vi "create.vi"(8 "error in (no error)":errorcluster, 10 "handle":i32, 11 "client":i32) -> (0 "error out":errorcluster, 3 "DatasetCreateStaging":refnum<class "DatasetCreateStaging.lvclass">)   [LabVIEW 2020, in "DatasetCreateStaging.lvclass"]
uses:
  DatasetCreateStaging.lvclass
  DatasetCreateStaging.lvclass/DatasetCreateStaging.ctl
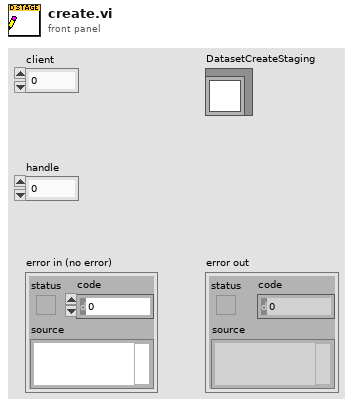
[diagram p1: front panel]
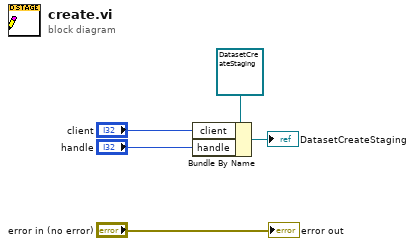
[diagram p0: block diagram]
diagram:
  n1 = Bundle By Name(cluster=refnum<class "DatasetCreateStaging.lvclass"> refnum ("DatasetCreateStaging in"), "client"="client", "handle"="handle") -> (→"DatasetCreateStaging":refnum<class "DatasetCreateStaging.lvclass">)
  "error out" <- "error in (no error)"
